vi "DFD FXP Set Quantizer.vi"   [LabVIEW 2017, in "NI_DigFilterLicensed.lvlib"]
doc: "Sets a quantizer or quantizers in a fixed-point filter. You must manually select the polymorphic instance you want to use."
uses:
  <vilib>/addons/Digital Filter Design/NI_DigFilterLicensed.lvlib
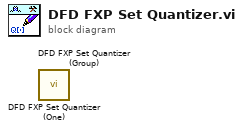
[diagram p0: block diagram]
diagram:
  n1 = call <vilib>:"DFD FXP Set Quantizer (One).vi"() -> ()  [unwired: 10 in, 2 out]
  n2 = call <vilib>:"DFD FXP Set Quantizer (Group).vi"() -> ()  [unwired: 10 in, 2 out]
